vi "ModuleStates.vi"() -> (1 "Module States":cluster{"Meters":dbl, "ROTATION":T1}[](array[cluster]) {"ROTATION"."SIN" format="%13.4f"; "ROTATION"."COS" format="%13.4f"; "ROTATION"."VALUE" format="%13.4f"}, 3 "Module Positions":T2[](array[typedef]) {"Angle"."SIN" format="%13.4f"; "Angle"."COS" format="%13.4f"; "Angle"."VALUE" format="%13.4f"})   [LabVIEW 2023]
uses:
  <vilib>/Rock Robotics/WPI/ThirdParty/JAS_Junk/TrajLib/Trajectory_Library.lvlib
  <vilib>/Rock Robotics/WPI/ThirdParty/JAS_Junk/TrajLib/TypeDef/ROTATION2D.ctl
  <vilib>/Rock Robotics/WPI/ThirdParty/JAS_Junk/TrajLib/TypeDef/SWERVE_DRIVE_MODULE_STATE.ctl
  <vilib>/Rock Robotics/WPI/ThirdParty/JAS_Junk/TrajLib/TypeDef/SWERVE_DRIVE_MODULE_POSITION.ctl
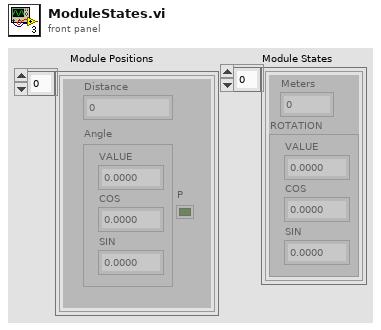
[diagram p1: front panel]
types:
  T1 = typedef "Trajectory_Library.lvlib/ROTATION2D.ctl" = cluster{"VALUE":dbl, "COS":dbl, "SIN":dbl}
  T2 = typedef "Trajectory_Library.lvlib/SWERVE_DRIVE_MODULE_POSITION.ctl" = cluster{"Distance":dbl, "Angle":T1, "P":bool}
  T3 = typedef "WPI_MotorControlDeviceRef.ctl" = cluster{"DeviceStatus":errorcluster, "Type":T4, "PWM":cluster{"PWM Channel":T5, "DeadBand":T6}, "CAN":cluster{"Device Number":u8, "SetOutput VI Ref":variant, "GetOutput VI Ref":variant, "Enable VI Ref":variant, "Disable VI Ref":variant, "Data":variant}, "Invert":bool, "DIO PWM":cluster{"PWM \"Enable\" Channel":T5, "DIOChannel":T7, "PWM Rate":dbl}}
  T4 = typedef "WPI_MotorControlType.ctl" = enum16{"PWM", "CAN", "DIO PWM"}
  T5 = typedef "FPGA_DIOPWMChannel.ctl" = enum8{"PWM 0", "PWM 1", "PWM 2", "PWM 3", "PWM 4", "PWM 5", "PWM 6", "PWM 7", "PWM 8", "PWM 9", "PWM MXP 0", "PWM MXP 1", "PWM MXP 2", "PWM MXP 3", "PWM MXP 4", "PWM MXP 5", "PWM MXP 6", "PWM MXP 7", "PWM MXP 8", "PWM MXP 9", "Invalid"}
  T6 = typedef "WPI_PWMDeadband.ctl" = cluster{"Name":string, "maxPositivePwm":i32, "minPositivePwm":i32, "centerPwm":i32, "maxNegativePwm":i32, "minNegativePwm":i32, "angularRange":u16}
  T7 = typedef "FPGA_DIOChannel.ctl" = enum8{"DIO 0", "DIO 1", "DIO 2", "DIO 3", "DIO 4", "DIO 5", "DIO 6", "DIO 7", "DIO 8", "DIO 9", "DIO MXP 0", "DIO MXP 1", "DIO MXP 2", "DIO MXP 3", "DIO MXP 4", "DIO MXP 5", "DIO MXP 6", "DIO MXP 7", "DIO MXP 8", "DIO MXP 9", "DIO MXP 10", "DIO MXP 11", "DIO MXP 12", "DIO MXP 13", "DIO MXP 14", "DIO MXP 15", "SPI Port CS1", "SPI Port CS2", "SPI Port CS3", "SPI Port MISO", "SPI Port MOSI", "Invalid"}
  T8 = typedef "Trajectory_Library.lvlib/SWERVE_DRIVE_MODULE_STATE.ctl" = cluster{"Speed":dbl, "Angle":T1}
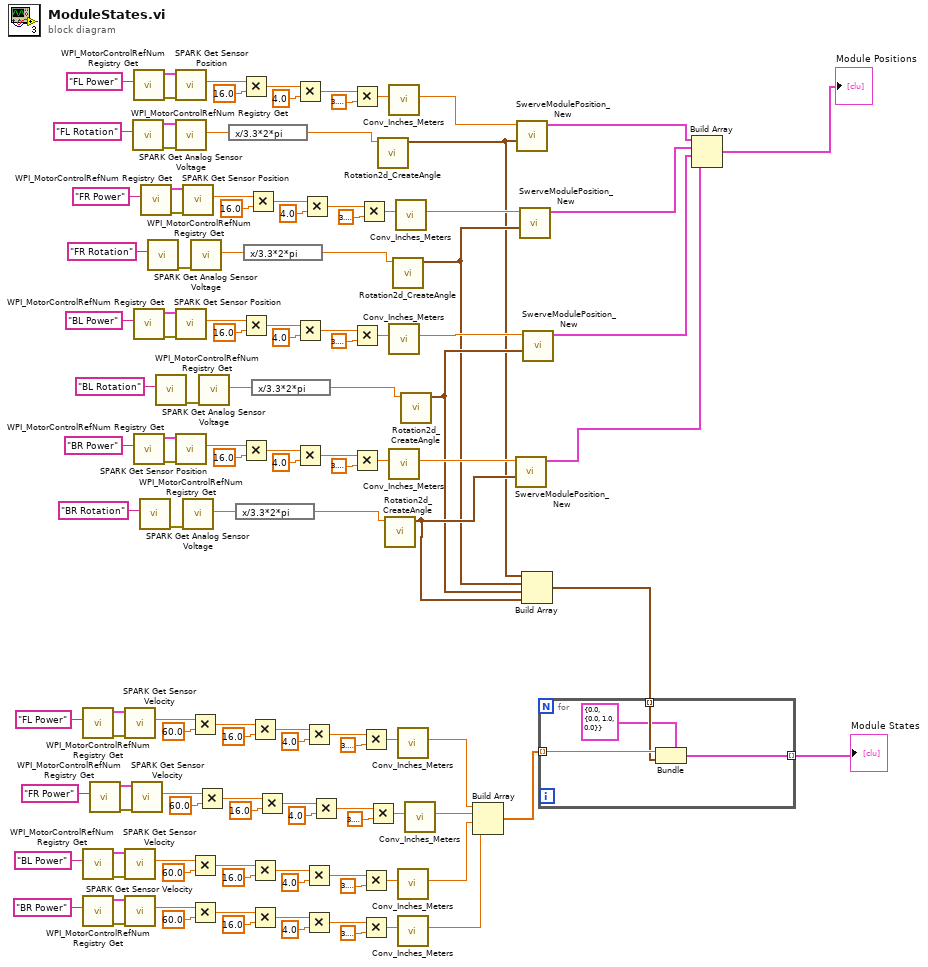
[diagram p0: block diagram]
diagram:
  n1 = call <vilib>:"WPI_MotorControlRefNum Registry Get.vi"("refnum name"="FL Power") -> ("error out"=w124:errorcluster, "MotorControlDevRef"=w123:T3)  [unwired: 9 in]
  n2 = call <vilib>:"WPI_MotorControlRefNum Registry Get.vi"("refnum name"="BL Power") -> ("error out"=w100:errorcluster, "MotorControlDevRef"=w99:T3)  [unwired: 9 in]
  n3 = call <vilib>:"WPI_MotorControlRefNum Registry Get.vi"("refnum name"="BR Power") -> ("error out"=w79:errorcluster, "MotorControlDevRef"=w80:T3)  [unwired: 9 in]
  n4 = call <vilib>:"WPI_MotorControlRefNum Registry Get.vi"("refnum name"="FR Power") -> ("error out"=w103:errorcluster, "MotorControlDevRef"=w104:T3)  [unwired: 9 in]
  n5 = call <vilib>:"SPARK Get Sensor Velocity.vi"("error in (no error)"=w124, "MotorControlDevRef in"=w123) -> ("Sensor Velocity"=w114:dbl)  [unwired: 6 in, 3 out]
  n6 = call <vilib>:"SPARK Get Sensor Velocity.vi"("error in (no error)"=w100, "MotorControlDevRef in"=w99) -> ("Sensor Velocity"=w90:dbl)  [unwired: 6 in, 3 out]
  n7 = call <vilib>:"SPARK Get Sensor Velocity.vi"("error in (no error)"=w79, "MotorControlDevRef in"=w80) -> ("Sensor Velocity"=w89:dbl)  [unwired: 6 in, 3 out]
  n8 = call <vilib>:"SPARK Get Sensor Velocity.vi"("error in (no error)"=w103, "MotorControlDevRef in"=w104) -> ("Sensor Velocity"=w113:dbl)  [unwired: 6 in, 3 out]
  n9 = call <vilib>:"WPI_MotorControlRefNum Registry Get.vi"("refnum name"="FL Rotation") -> ("error out"=w30:errorcluster, "MotorControlDevRef"=w29:T3)  [unwired: 9 in]
  n10 = call <vilib>:"WPI_MotorControlRefNum Registry Get.vi"("refnum name"="FL Power") -> ("error out"=w67:errorcluster, "MotorControlDevRef"=w66:T3)  [unwired: 9 in]
  n11 = call <vilib>:"WPI_MotorControlRefNum Registry Get.vi"("refnum name"="BL Power") -> ("error out"=w63:errorcluster, "MotorControlDevRef"=w62:T3)  [unwired: 9 in]
  n12 = call <vilib>:"WPI_MotorControlRefNum Registry Get.vi"("refnum name"="BR Power") -> ("error out"=w61:errorcluster, "MotorControlDevRef"=w60:T3)  [unwired: 9 in]
  n13 = call <vilib>:"WPI_MotorControlRefNum Registry Get.vi"("refnum name"="BR Rotation") -> ("error out"=w11:errorcluster)  [unwired: 9 in, 1 out]
  n14 = call <vilib>:"WPI_MotorControlRefNum Registry Get.vi"("refnum name"="FR Power") -> ("error out"=w65:errorcluster, "MotorControlDevRef"=w64:T3)  [unwired: 9 in]
  n15 = call <vilib>:"WPI_MotorControlRefNum Registry Get.vi"("refnum name"="FR Rotation") -> ("error out"=w21:errorcluster)  [unwired: 9 in, 1 out]
  n16 = call <vilib>:"WPI_MotorControlRefNum Registry Get.vi"("refnum name"="BL Rotation") -> ("error out"=w18:errorcluster)  [unwired: 9 in, 1 out]
  n17 = call <vilib>:"SPARK Get Sensor Position.vi"("error in (no error)"=w67, "MotorControlDevRef in"=w66) -> ("Sensor Position"=w32:dbl)  [unwired: 6 in, 3 out]
  n18 = call <vilib>:"SPARK Get Analog Sensor Voltage.vi"("error in (no error)"=w30, "MotorControlDevRef in"=w29) -> ("Analog Sensor Voltage"=w28:dbl)  [unwired: 6 in, 3 out]
  n19 = call <vilib>:"SPARK Get Sensor Position.vi"("error in (no error)"=w63, "MotorControlDevRef in"=w62) -> ("Sensor Position"=w46:dbl)  [unwired: 6 in, 3 out]
  n20 = call <vilib>:"SPARK Get Sensor Position.vi"("error in (no error)"=w61, "MotorControlDevRef in"=w60) -> ("Sensor Position"=w53:dbl)  [unwired: 6 in, 3 out]
  n21 = call <vilib>:"SPARK Get Sensor Position.vi"("error in (no error)"=w65, "MotorControlDevRef in"=w64) -> ("Sensor Position"=w39:dbl)  [unwired: 6 in, 3 out]
  n22 = call <vilib>:"SPARK Get Analog Sensor Voltage.vi"("error in (no error)"=w11) -> ("Analog Sensor Voltage"=w12:dbl)  [unwired: 7 in, 3 out]
  n23 = Multiply(x=w114, y=60.0) -> (x*y=w117:dbl)
  n24 = Multiply(x=w90, y=60.0) -> (x*y=w93:dbl)
  n25 = Multiply(x=w89, y=60.0) -> (x*y=w86:dbl)
  n26 = call <vilib>:"SPARK Get Analog Sensor Voltage.vi"("error in (no error)"=w21) -> ("Analog Sensor Voltage"=w22:dbl)  [unwired: 7 in, 3 out]
  n27 = Multiply(x=w113, y=60.0) -> (x*y=w110:dbl)
  n28 = call <vilib>:"SPARK Get Analog Sensor Voltage.vi"("error in (no error)"=w18) -> ("Analog Sensor Voltage"=w17:dbl)  [unwired: 7 in, 3 out]
  n29 = expression code="x/3.3*2*pi"(w28) -> (w27:dbl)
  n30 = expression code="x/3.3*2*pi"(w12) -> (w13:dbl)
  n31 = Multiply(x=w32, y=16.0) -> (x*y=w34:dbl)
  n32 = Multiply(x=w46, y=16.0) -> (x*y=w48:dbl)
  n33 = Multiply(x=w53, y=16.0) -> (x*y=w58:dbl)
  n34 = expression code="x/3.3*2*pi"(w22) -> (w23:dbl)
  n35 = Multiply(x=w39, y=16.0) -> (x*y=w44:dbl)
  n36 = Multiply(x=w117, y=16.0) -> (x*y=w116:dbl)
  n37 = Multiply(x=w93, y=16.0) -> (x*y=w92:dbl)
  n38 = Multiply(x=w86, y=16.0) -> (x*y=w87:dbl)
  n39 = expression code="x/3.3*2*pi"(w17) -> (w16:dbl)
  n40 = Multiply(x=w110, y=16.0) -> (x*y=w111:dbl)
  n41 = Multiply(x=w34, y=4.0) -> (x*y=w36:dbl)
  n42 = Multiply(x=w48, y=4.0) -> (x*y=w50:dbl)
  n43 = Multiply(x=w58, y=4.0) -> (x*y=w56:dbl)
  n44 = Multiply(x=w44, y=4.0) -> (x*y=w42:dbl)
  n45 = Multiply(x=w116, y=4.0) -> (x*y=w115:dbl)
  n46 = Multiply(x=w92, y=4.0) -> (x*y=w91:dbl)
  n47 = Multiply(x=w87, y=4.0) -> (x*y=w88:dbl)
  n48 = Multiply(x=w111, y=4.0) -> (x*y=w112:dbl)
  n49 = Multiply(x=w36, y=3.141592653589793) -> (x*y=w38:dbl)
  n50 = Multiply(x=w50, y=3.141592653589793) -> (x*y=w52:dbl)
  n51 = Multiply(x=w56, y=3.141592653589793) -> (x*y=w54:dbl)
  n52 = Multiply(x=w42, y=3.141592653589793) -> (x*y=w40:dbl)
  n53 = Multiply(x=w115, y=3.141592653589793) -> (x*y=w118:dbl)
  n54 = Multiply(x=w91, y=3.141592653589793) -> (x*y=w94:dbl)
  n55 = Multiply(x=w88, y=3.141592653589793) -> (x*y=w85:dbl)
  n56 = Multiply(x=w112, y=3.141592653589793) -> (x*y=w109:dbl)
  n57 = call <vilib>:"Rotation2d_CreateAngle.vi"("Angle"=w27) -> ("ROTATION"=w2:T1)  [unwired: 10 in]
  n58 = call <vilib>:"Rotation2d_CreateAngle.vi"("Angle"=w13) -> ("ROTATION"=w5:T1)  [unwired: 10 in]
  n59 = call <vilib>:"Conv_Inches_Meters.vi"("INCH"=w38) -> ("Meters"=w26:dbl)  [unwired: 10 in]
  n60 = call <vilib>:"Conv_Inches_Meters.vi"("INCH"=w52) -> ("Meters"=w14:dbl)  [unwired: 10 in]
  n61 = call <vilib>:"Conv_Inches_Meters.vi"("INCH"=w54) -> ("Meters"=w9:dbl)  [unwired: 10 in]
  n62 = call <vilib>:"Rotation2d_CreateAngle.vi"("Angle"=w23) -> ("ROTATION"=w3:T1)  [unwired: 10 in]
  n63 = call <vilib>:"Conv_Inches_Meters.vi"("INCH"=w40) -> ("Meters"=w15:dbl)  [unwired: 10 in]
  n64 = call <vilib>:"Conv_Inches_Meters.vi"("INCH"=w118) -> ("Meters"=w76:dbl)  [unwired: 10 in]
  n65 = call <vilib>:"Conv_Inches_Meters.vi"("INCH"=w94) -> ("Meters"=w74:dbl)  [unwired: 10 in]
  n66 = call <vilib>:"Conv_Inches_Meters.vi"("INCH"=w85) -> ("Meters"=w73:dbl)  [unwired: 10 in]
  n67 = call <vilib>:"Rotation2d_CreateAngle.vi"("Angle"=w16) -> ("ROTATION"=w4:T1)  [unwired: 10 in]
  n68 = call <vilib>:"Conv_Inches_Meters.vi"("INCH"=w109) -> ("Meters"=w75:dbl)  [unwired: 10 in]
  n69 = Build Array(w76, w75, w74, w73) -> (w77:dbl[])
  n70 = call <vilib>:"SwerveModulePosition_New.vi"("ROTATION"=w5, "Distance"=w9) -> ("SWERVE_DRIVE_MODULE_POSITION"=w6:T2)  [unwired: 9 in]
  n71 = call <vilib>:"SwerveModulePosition_New.vi"("ROTATION"=w2, "Distance"=w26) -> ("SWERVE_DRIVE_MODULE_POSITION"=w25:T2)  [unwired: 9 in]
  n72 = call <vilib>:"SwerveModulePosition_New.vi"("ROTATION"=w3, "Distance"=w15) -> ("SWERVE_DRIVE_MODULE_POSITION"=w8:T2)  [unwired: 9 in]
  n73 = Build Array(w2, w3, w4, w5) -> (w1:T1[])
  n74 = call <vilib>:"SwerveModulePosition_New.vi"("ROTATION"=w4, "Distance"=w14) -> ("SWERVE_DRIVE_MODULE_POSITION"=w7:T2)  [unwired: 9 in]
  n75 = for {
    tunnel: w77 -> [w129] mode=indexing
    tunnel: w1 -> [w128] mode=indexing
    tunnel: [w127] -> w72 mode=indexing
    n76 = Bundle(cluster=T8 {"Speed"=0.0, "Angle"={"VALUE"=0.0, "COS"=1.0, "SIN"=0.0}} ("SWERVE_DRIVE_MODULE_STATE"), "Speed"=w129, "Angle"=w128) -> (w127:T8)
  }
  "Module States" <- w72
  n77 = Build Array(w25, w8, w7, w6) -> (→"Module Positions":T2[])
